vi "HOLD.vi"(0 "VISA resource name":refnum<visa-resource-name>, 1 "Timeout (s)":string, 2 "Message Line 1":string, 3 "Message Line 2":string, 4 "Command Terminator":bool=TRUE, 5 "error in (no error)":errorcluster) -> (14 "VISA resource name out":refnum<visa-resource-name>, 15 "Command Output":string="\r", 17 "Error Message":string, 18 "Error Code":i32, 19 "error out":errorcluster)   [LabVIEW 2010, in "VITREK V7X.lvlib"]
doc: "Configures the <b>HOLD</b> input.\n\n<b>Note:</b> please refer to the instrument manual for the <b>HOLD</b> input specification."
uses:
  VITREK V7X.lvlib
panel:
  # "Yes\n\nNo"
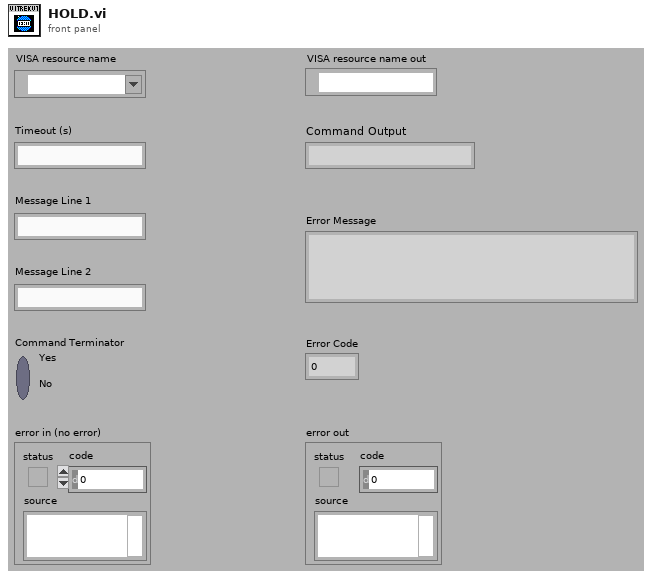
[diagram p1: front panel]
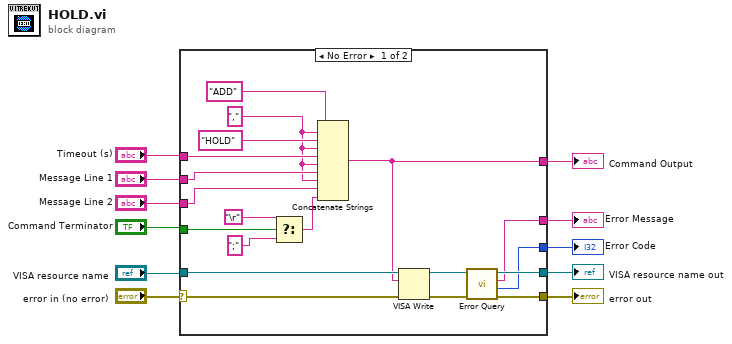
[diagram p0: block diagram]
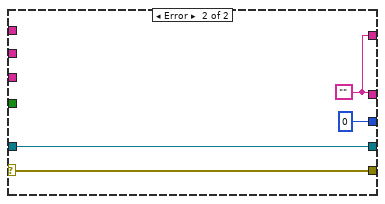
[diagram p2: hidden frame]
diagram:
  n1 = case shown="No Error" "error in (no error)" {
    selector: "error in (no error)" -> [w25 w33]
    tunnel: "VISA resource name" -> [w30 w34]
    tunnel: [w23 w31] -> w10
    tunnel: [w27 w34] -> w9
    tunnel: [w26 w33] -> w8
    tunnel: "Timeout (s)" -> [w18 _]
    tunnel: "Command Terminator" -> [w22 _]
    tunnel: "Message Line 1" -> [w17 _]
    tunnel: "Message Line 2" -> [w15 _]
    tunnel: [w13 0] -> w2
    tunnel: [w12 w31] -> w1
    frame No Error {
      w16 = ","
      n2 = Select(t="\r", s=w22, f=";") -> (s? t:f=w14:string)
      n3 = Concatenate Strings("ADD", w16, "HOLD", w16, w18, w16, w17, w16, w15, w14) -> (w23:string)
      n4 = VISA Write(VISA resource name=w30, write buffer=w23, error in (no error)=w25) -> (VISA resource name out=w29:refnum<visa-resource-name>, error out=w28:errorcluster)  [unwired: 1 out]
      n5 = call "Error Query.vi"("error in (no error)"=w28, "VISA resource name"=w29) -> ("error out"=w26:errorcluster, "Error Code"=w13:i32, "Error Message"=w12:string, "VISA resource name out"=w27:refnum<visa-resource-name>)  [unwired: 6 in]
    }
    frame Error {
      w31 = ""
    }
  }
  "VISA resource name out" <- w9
  "error out" <- w8
  "Command Output" <- w10
  "Error Code" <- w2
  "Error Message" <- w1
